vi "Do.vi"(7 "Mediated Asynchronous Actor":refnum<class "Mediated Asynchronous Actor.lvclass">, 8 "error in (no error)":errorcluster, 11 "Launch Client Handler Actor Msg in":refnum<class "Launch Client Handler Actor Msg.lvclass">) -> (0 "error out":errorcluster, 3 "Launch Client Handler Actor Msg out":refnum<class "Launch Client Handler Actor Msg.lvclass">, 5 "Mediated Asynchronous Actor out":refnum<class "Mediated Asynchronous Actor.lvclass">)   [LabVIEW 2016, in "Stream Mediator.lvlib" / "Launch Client Handler Actor Msg.lvclass"]
doc: "--\nCopyright © 2017 Composed SystemsI All rights reserved.\n\nAuthor: Jon McBee <jon.mcbee@composed.io>\n\nThis library is provided \"AS IS\" ,WITHOUT WARRANTIES OR\nCONDITIONS OF ANY KIND, either express or implied.\n\nComposed Systems -- composed.io\n\nStream 0.0.1.1\nJon McBee - Composed Systems\nCopyright (c) 2017, Composed Systems"
uses:
  <userlib>/Composed Systems/Stream/Mediator/Classes/Websocket Server Actor/Websocket Server Msgs/Launch Client Handler Actor Msg/Launch Client Handler Actor Msg.lvclass
  <userlib>/Composed Systems/Stream/Mediator/Classes/Mediated Asynchronous Actor/Mediated Asynchronous Actor.lvclass
  <userlib>/Composed Systems/Stream/Mediator/Classes/Websocket Server Actor/Websocket Server/Websocket Server.lvclass
  C:/Program Files (x86)/National Instruments/LabVIEW 2016/user.lib/Composed Systems/Stream/Mediator/Classes/Mediated Asynchronous Actor/Mediated Asynchronous Actor.lvclass
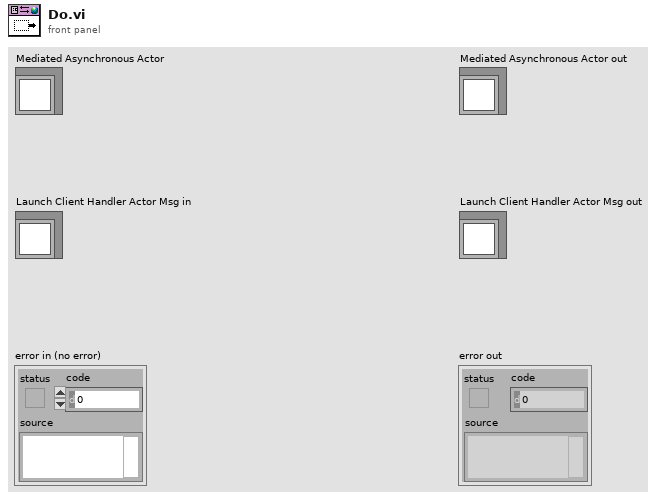
[diagram p1: front panel]
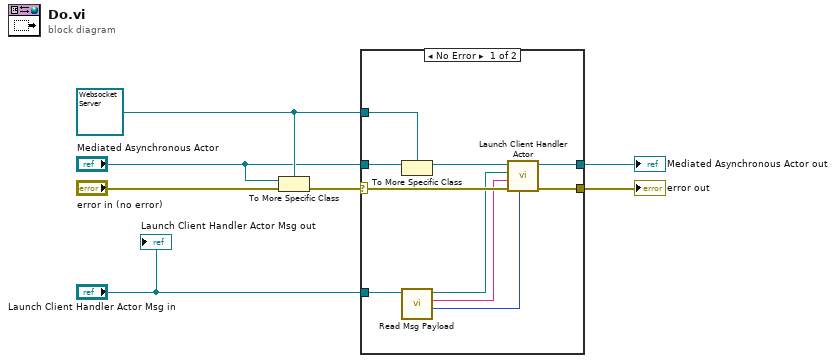
[diagram p0: block diagram]
diagram:
  w5 = refnum<class "Websocket Server.lvclass"> refnum ("Websocket Server.lvclass")
  n1 = To More Specific Class(target class=w5, reference="Mediated Asynchronous Actor", error in="error in (no error)") -> (error out=w7:errorcluster)  [unwired: 1 out]
  n2 = case shown="No Error" w7 {
    selector: w7 -> [w14 w18]
    tunnel: w5 -> [w17 _]
    tunnel: "Mediated Asynchronous Actor" -> [w16 w19]
    tunnel: "Launch Client Handler Actor Msg in" -> [w11 _]
    tunnel: [w13 w19] -> w3
    tunnel: [w12 w18] -> w1
    frame No Error {
      n3 = To More Specific Class(target class=w17, reference=w16) -> (specific class reference=w15:refnum<class "Websocket Server.lvclass">)  [unwired: 1 in, 1 out]
      n4 = call <userlib>:"Read Msg Payload.vi"("Launch Client Handler Actor Msg in"=w11) -> ("timeout ms (5000)"=w8:i32, "Remote Address"=w9:string, "WebSocket Connection in"=w10:refnum<k5>)  [unwired: 7 in, 1 out]
      n5 = call <userlib>:"Launch Client Handler Actor.vi"("timeout ms (5000)"=w8, "error in (no error)"=w14, "Remote Address"=w9, "WebSocket Connection in"=w10, "Websocket Server in"=w15) -> ("error out"=w12:errorcluster, "Websocket Server out"=w13:refnum<class "Websocket Server.lvclass">)  [unwired: 5 in]
    }
    frame Error {
    }
  }
  "error out" <- w1
  "Mediated Asynchronous Actor out" <- w3
  "Launch Client Handler Actor Msg out" <- "Launch Client Handler Actor Msg in"
